vi "UarmTestRead.vi"() -> ()   [LabVIEW 2017]
panel:
  in  "stop":bool
  in  "GCode Command":string
  in  "error in":errorcluster
  out "error out":errorcluster
  in  "VISA Refnum in":refnum<visa-resource-name>="ASRL1::INSTR"
  out "read buffer":string
  in  "Sen":bool
  # "#n G0 X100 Y100 Z100 F1000\\n"
  # "#n M2400 S0\\n"
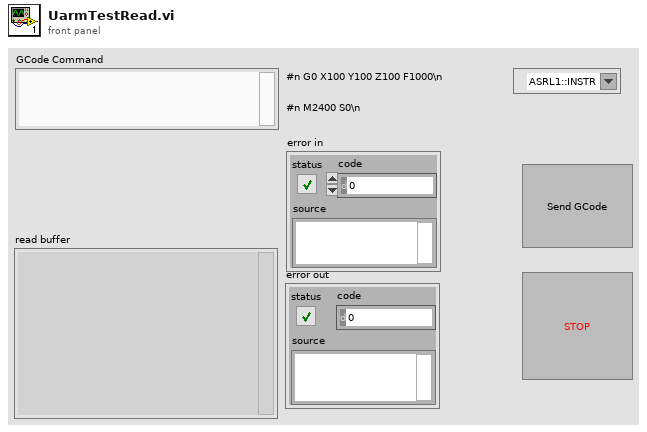
[diagram p1: front panel]
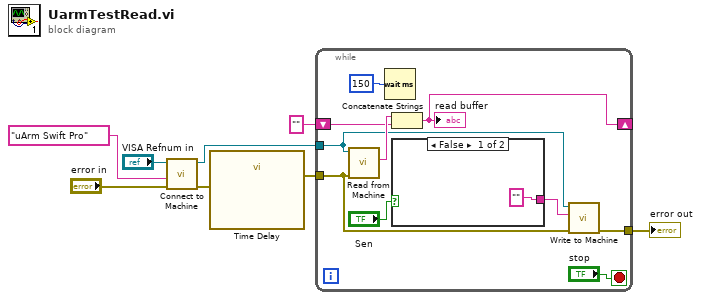
[diagram p0: block diagram]
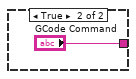
[diagram p2: hidden frame]
diagram:
  n1 = call "Connect to Machine .vi"(8:"error in", "Firmware"="uArm Swift Pro", "Machine In"="VISA Refnum in") -> ("error out"=w7:errorcluster, "Machine Out"=w3:refnum<visa-resource-name>)  [unwired: 6 in, 1 out]
  n2 = call "Time Delay"("error in (no error)"=w7) -> ("error out"=w4:errorcluster)  [unwired: 10 in]
  n3 = while {
    tunnel: w3 -> [w11]
    tunnel: w4 -> [w12]
    tunnel: [w16] -> w2
    shift-right: [w10] -> _
    shift-left: "" -> [w13]
    stop <- "stop" stop-if-true
    n4 = call "Read from Machine.vi"("error in (no error)"=w12, "Machine In"=w11) -> ("read buffer"=w14:string)  [unwired: 7 in, 2 out]
    n5 = Wait (ms)(milliseconds to wait=u32 150) -> ()  [unwired: 1 out]
    n6 = Concatenate Strings(w14, w13) -> (w10:string)
    "read buffer" <- w10
    n7 = case shown="False" "Sen" {
      tunnel: ["" ("Write Buffer") "GCode Command"] -> w9
      frame False {
      }
      frame True {
      }
    }
    n8 = call "Write to Machine .vi"("error in (no error)"=w12, "G-Code String In"=w9, "Machine In"=w11) -> ("error out"=w16:errorcluster)  [unwired: 7 in, 1 out]
  }
  "error out" <- w2
